vi "EminemNetworking.vi"(8 "error in (no error)":errorcluster) -> (0 "error out":errorcluster)   [LabVIEW 2023]
uses:
  EminemGlobals.vi
  <vilib>/Rock Robotics/Network Tables/NT Write Number.vi
  <vilib>/Rock Robotics/Network Tables/NT Write Boolean.vi
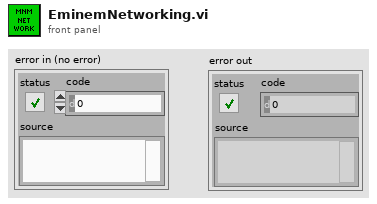
[diagram p1: front panel]
types:
  T1 = typedef "EminemStatesEnum.ctl" = enum16{"0-Init", "1-WaitForCmd", "2-Cancel", "3-ShootStart", "4-ShootRev", "5-RevUpStart", "6-ShootStartFeed&Timer", "7-ShootTimerOrSensorDone", "8-ShootDone", "9-AmpStart", "10-AmpUpToSpd?", "11-AmpStartFeed&Timer", "12-AmpTimerOrSensorDone", "13-AmpDone", "14-RevUpGetCmd"}
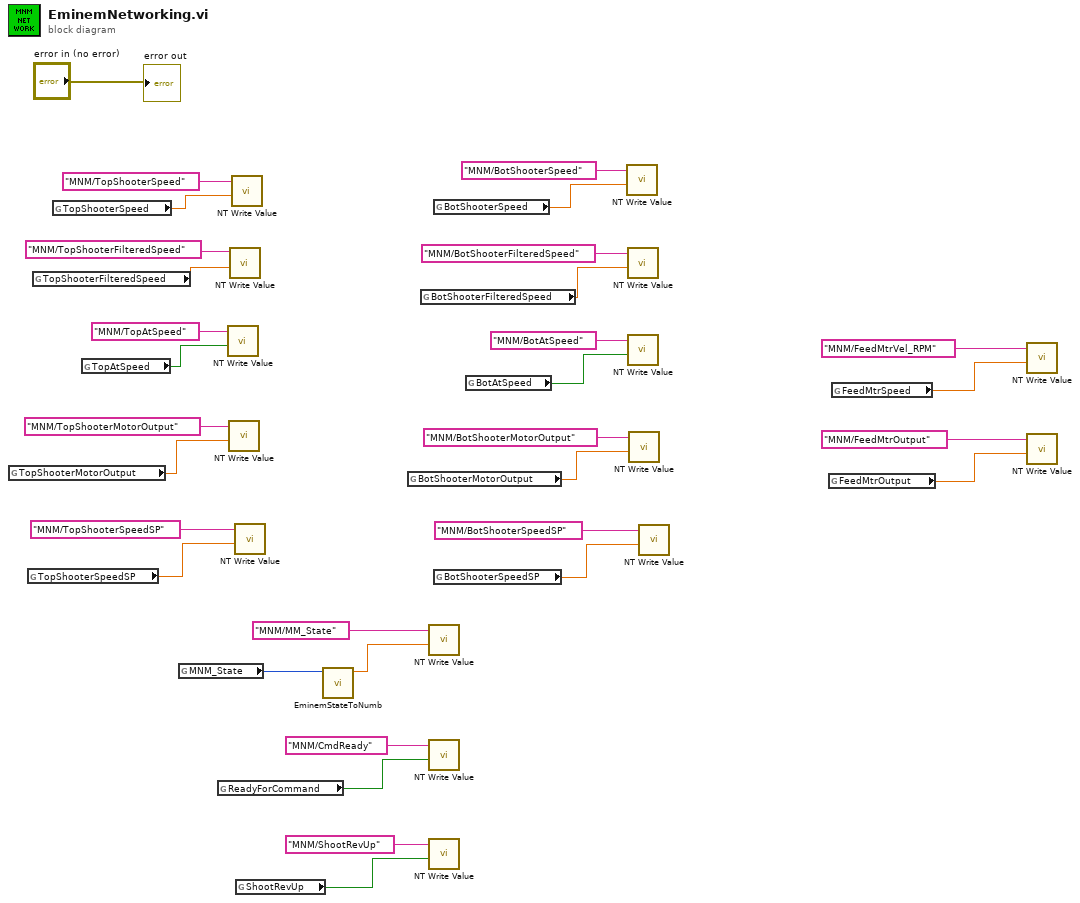
[diagram p0: block diagram]
diagram:
  n1 = global read "EminemGlobals.vi" "TopShooterMotorOutput"() -> (w16:dbl)
  n2 = global read "EminemGlobals.vi" "TopShooterSpeedSP"() -> (w3:dbl)
  n3 = global read "EminemGlobals.vi" "TopShooterFilteredSpeed"() -> (w22:dbl)
  n4 = global read "EminemGlobals.vi" "TopShooterSpeed"() -> (w21:dbl)
  n5 = global read "EminemGlobals.vi" "TopAtSpeed"() -> (w20:bool)
  n6 = global read "EminemGlobals.vi" "MNM_State"() -> (w11:T1)
  n7 = global read "EminemGlobals.vi" "ReadyForCommand"() -> (w14:bool)
  n8 = call-poly <vilib>:"NT Write Value.vi"("value"=w20, "name"="MNM/TopAtSpeed") -> ()  [unwired: 9 in, 1 out]
  n9 = call-poly <vilib>:"NT Write Value.vi"("value"=w16, "name"="MNM/TopShooterMotorOutput") -> ()  [unwired: 9 in, 1 out]
  n10 = call-poly <vilib>:"NT Write Value.vi"("value"=w22, "name"="MNM/TopShooterFilteredSpeed") -> ()  [unwired: 9 in, 1 out]
  n11 = call-poly <vilib>:"NT Write Value.vi"("value"=w21, "name"="MNM/TopShooterSpeed") -> ()  [unwired: 9 in, 1 out]
  n12 = call-poly <vilib>:"NT Write Value.vi"("value"=w3, "name"="MNM/TopShooterSpeedSP") -> ()  [unwired: 9 in, 1 out]
  n13 = global read "EminemGlobals.vi" "ShootRevUp"() -> (w5:bool)
  n14 = call "EminemStateToNumb.vi"("Eminim_state"=w11) -> ("StateNumber"=w9:dbl)  [unwired: 10 in]
  n15 = global read "EminemGlobals.vi" "BotShooterMotorOutput"() -> (w15:dbl)
  n16 = global read "EminemGlobals.vi" "BotShooterFilteredSpeed"() -> (w18:dbl)
  n17 = call-poly <vilib>:"NT Write Value.vi"("value"=w9, "name"="MNM/MM_State") -> ()  [unwired: 9 in, 1 out]
  n18 = call-poly <vilib>:"NT Write Value.vi"("value"=w14, "name"="MNM/CmdReady") -> ()  [unwired: 9 in, 1 out]
  n19 = call-poly <vilib>:"NT Write Value.vi"("value"=w5, "name"="MNM/ShootRevUp") -> ()  [unwired: 9 in, 1 out]
  n20 = global read "EminemGlobals.vi" "BotShooterSpeed"() -> (w19:dbl)
  n21 = global read "EminemGlobals.vi" "BotShooterSpeedSP"() -> (w1:dbl)
  n22 = global read "EminemGlobals.vi" "BotAtSpeed"() -> (w17:bool)
  n23 = call-poly <vilib>:"NT Write Value.vi"("value"=w19, "name"="MNM/BotShooterSpeed") -> ()  [unwired: 9 in, 1 out]
  n24 = call-poly <vilib>:"NT Write Value.vi"("value"=w18, "name"="MNM/BotShooterFilteredSpeed") -> ()  [unwired: 9 in, 1 out]
  n25 = call-poly <vilib>:"NT Write Value.vi"("value"=w17, "name"="MNM/BotAtSpeed") -> ()  [unwired: 9 in, 1 out]
  n26 = call-poly <vilib>:"NT Write Value.vi"("value"=w15, "name"="MNM/BotShooterMotorOutput") -> ()  [unwired: 9 in, 1 out]
  n27 = call-poly <vilib>:"NT Write Value.vi"("value"=w1, "name"="MNM/BotShooterSpeedSP") -> ()  [unwired: 9 in, 1 out]
  n28 = global read "EminemGlobals.vi" "FeedMtrOutput"() -> (w12:dbl)
  n29 = global read "EminemGlobals.vi" "FeedMtrSpeed"() -> (w7:dbl)
  n30 = call-poly <vilib>:"NT Write Value.vi"("value"=w7, "name"="MNM/FeedMtrVel_RPM") -> ()  [unwired: 9 in, 1 out]
  n31 = call-poly <vilib>:"NT Write Value.vi"("value"=w12, "name"="MNM/FeedMtrOutput") -> ()  [unwired: 9 in, 1 out]
  "error out" <- "error in (no error)"
